vi "Create Session(s).vi"   [LabVIEW 2020, in "MeasurementLink niDCPower.lvlib"]
uses:
  MeasurementLink niDCPower.lvlib
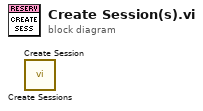
[diagram p0: block diagram]
diagram:
  n1 = call "Create Sessions.vi"() -> ()  [unwired: 8 in, 4 out]
  n2 = call "Create Session.vi"() -> ()  [unwired: 8 in, 4 out]
